vi "Download Trip File.vi"(8 "error in (no error)":errorcluster, 9 "Download Progress Ref":refnum<vi>, 10 "File Name":string, 11 "TCP Network Connection in":refnum<k5>) -> (0 "error out":errorcluster, 3 "File Name Out":string)   [LabVIEW 2019]
doc: "Author: Scott Hannahs <sth@magnet.fsu.edu>\nCopyright 2018 Florida State University, All rights reserved."
uses:
  TCP Functions/TCP Read Length and Value (U32).vi
  TCP Functions/TCP Read Length and Value (STR).vi
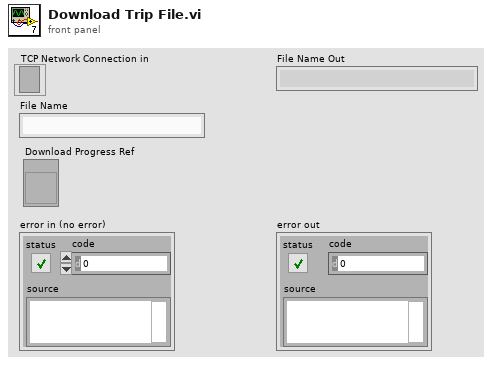
[diagram p1: front panel]
types:
  T1 = enum16{"open", "replace", "create", "open or create", "replace or create", "replace or create with confirmation"}
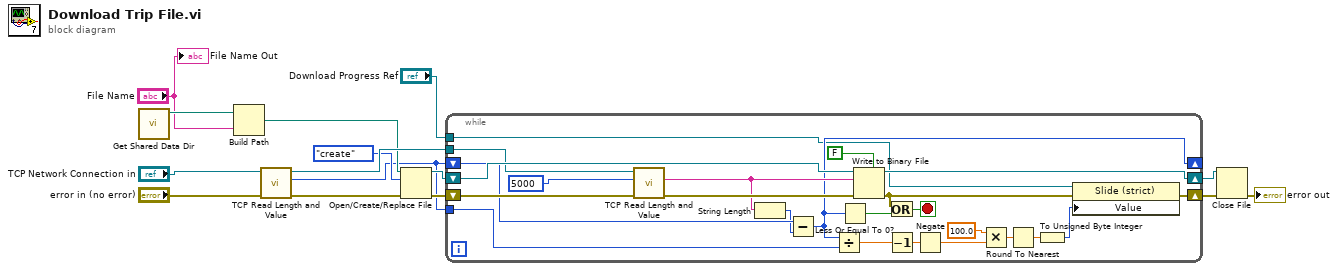
[diagram p0: block diagram]
diagram:
  n1 = call "Get Shared Data Dir.vi"() -> ("Data Directory Path"=w6:path)  [unwired: 2 in, 1 out]
  n2 = Build Path(base path=w6, name or relative path="File Name") -> (appended path=w11:path)
  n3 = call-poly "TCP Read Length and Value.vi"("error in (no error)"="error in (no error)", "TCP Network Connection in"="TCP Network Connection in") -> ("error out"=w13:errorcluster, "Output"=w2:u32, "TCP Network Connection out"=w12:refnum<k5>)  [unwired: 7 in]
  n4 = Open/Create/Replace File(file path (use dialog)=w11, error in=w13, operation (0:open)=T1."create") -> (refnum out=w9:refnum<file>, error out=w10:errorcluster)  [unwired: 3 in, 1 out]
  n5 = while {
    shift-right: [w16] -> w15
    shift-left: w10 -> [w38]
    shift-right: [w36] -> w14
    shift-left: w9 -> [w37]
    tunnel: w12 -> [w34]
    shift-right: [w27] -> _
    shift-left: w2 -> [w32]
    tunnel: w2 -> [w26]
    tunnel: "Download Progress Ref" -> [w18]
    stop <- w28 stop-if-true
    n6 = call-poly "TCP Read Length and Value.vi"("error in (no error)"=w38, "timeout ms (1000)"=5000, "TCP Network Connection in"=w34) -> ("error out"=w39:errorcluster, "Output"=w30:string)  [unwired: 6 in, 1 out]
    n7 = String Length(string=w30) -> (length=w31:i32)
    n8 = Subtract(x=w32, y=w31) -> (x-y=w27:u32)
    n9 = Divide(x=w27, y=w26) -> (x/y=w25:dbl)
    n10 = Less Or Equal To 0?(x=w27) -> (x <= 0?=w29:bool)
    n11 = Write to Binary File(file (use dialog)=w37, data=w30, error in=w39, 5:FALSE ("prepend array or string size? (T)")) -> (refnum out=w36:refnum<file>, error out=w17:errorcluster)  [unwired: 2 in, 1 out]
    n12 = Or(x=w17, y=w29) -> (x .or. y?=w28:bool)
    n13 = Decrement(x=w25) -> (x-1=w24:dbl)
    n14 = Negate(x=w24) -> (-x=w23:dbl)
    n15 = Multiply(x=100.0, y=w23) -> (x*y=w21:dbl)
    n16 = Round To Nearest(number=w21) -> (nearest integer value=w20:dbl)
    n17 = To Unsigned Byte Integer(number=w20) -> (unsigned 8bit integer=w19:u8)
    n18 = property class="Slide (strict)"(reference=w18, error in=w17, "Value"=w19) -> (error out=w16:errorcluster)  [unwired: 1 out]
  }
  n19 = Close File(refnum=w14, error in=w15) -> (error out=→"error out":errorcluster)  [unwired: 1 out]
  "File Name Out" <- "File Name"
